vi "Verify Repsonse.vi"(8 "error in (no error)":errorcluster, 11 "Sift Client in":refnum<class "Sift Client.lvclass">) -> (0 "error out":errorcluster, 3 "Sift Client out":refnum<class "Sift Client.lvclass">)   [LabVIEW 2024, in "Sift Client.lvlib" / "Sift Client.lvclass"]
uses:
  Sift Client.lvclass
  Sift Client.lvclass/Sift Client.ctl
  <userlib>/_OpenG.lib/error/error.llb/openg_error.lvlib
panel:
  out "Response":string
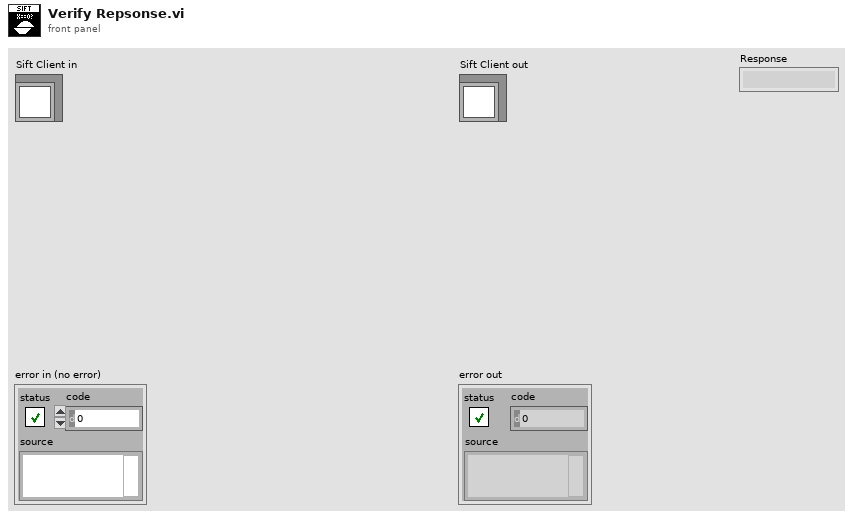
[diagram p1: front panel]
types:
  T1 = enum16{"Standard", "Buffered", "CRLF", "Immediate"}
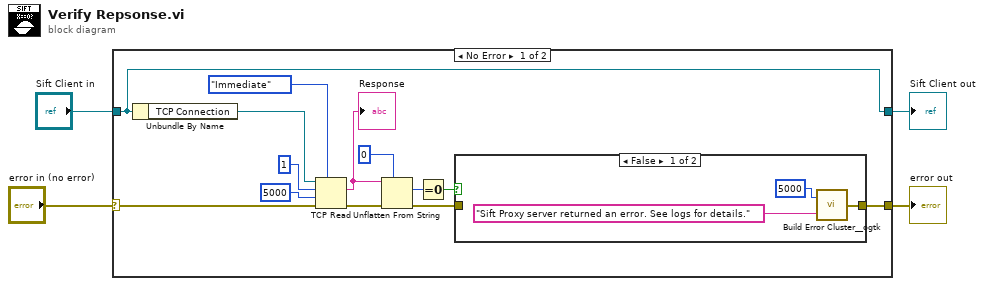
[diagram p0: block diagram]
diagram:
  n1 = case shown="No Error" "error in (no error)" {
    selector: "error in (no error)" -> [w13 w23]
    tunnel: [w7 w23] -> w3
    tunnel: [w14 w22] -> w1
    tunnel: "Sift Client in" -> [w14 w22]
    frame No Error {
      n2 = Unbundle By Name(w14) -> ("TCP Connection"=w17:refnum<k5>)
      n3 = TCP Read(connection ID=w17, bytes to read=1, error in (no error)=w13, 7:T1."Immediate" ("mode (standard)"), 9:5000 ("timeout ms (25000)")) -> (data out=w12:string, error out=w11:errorcluster)  [unwired: 1 out]
      "Response" <- w12
      n4 = Unflatten From String(type=u8 0, binary string=w12, error in (no error)=w11) -> (value=w9:u8, error out=w6:errorcluster)  [unwired: 2 in, 1 out]
      n5 = Equal To 0?(x=w9) -> (x = 0?=w8:bool)
      n6 = case shown="False" w8 {
        tunnel: [w20 w21] -> w7
        tunnel: w6 -> [_ w21]
        frame False {
          n7 = call <userlib>:"Build Error Cluster__ogtk.vi"("String to Prepend to source (\"\")"="Sift Proxy server returned an error. See logs for details.", "code"=5000) -> ("error out"=w20:errorcluster)
        }
        frame True {
        }
      }
    }
    frame Error {
    }
  }
  "error out" <- w3
  "Sift Client out" <- w1
